vi "Y Scale Name Label Text Write.vi"(4 "error in (no error)":errorcluster, 5 "Value":string, 6 "Container State":T3, 7 "Display State In":T1) -> (0 "error out":errorcluster, 3 "Display State Out":T1)   [LabVIEW 2017, in "2D Feather.xctl"]
uses:
  <vilib>/Math Plots/2D Math Plots/2D Feather/2D Feather XCtrl/2D Feather.xctl
  <vilib>/_xctls/Container State.ctl
  <vilib>/Math Plots/2D Math Plots/2D Feather/2D Feather XCtrl/State.ctl
  <vilib>/Math Plots/2D Math Plots/2D Feather/2D Feather/2D Feather.lvclass
  e:/builds/penguin/labview/branches/2017/dev/dist/vi.lib/Math Plots/2D Math Plots/2D Plot/2D Plot/2D Plot.lvclass
  <vilib>/Math Plots/2D Math Plots/2D Plot/Action String/2DMathPlot Ctrl Act Queue.ctl
  <vilib>/Math Plots/2D Math Plots/2D Plot/Action String/2DMathPlot Ctrl Act Cluster.ctl
  <vilib>/Math Plots/2D Math Plots/2D Plot/Action String/2DMathPlot State Class.ctl
  <vilib>/Math Plots/2D Math Plots/2D Plot/2D Plot/2D Plot.lvclass
  <vilib>/_xctls/XControlSupport.lvlib
panel:
  # "Replace the Value Control below with a Control of desired type.\nDo not remove this Control or the others from the connector pane.\nDo not change the connector pane pattern.\nThe Value control should always be the third terminal from top on the input side in the connector pane."
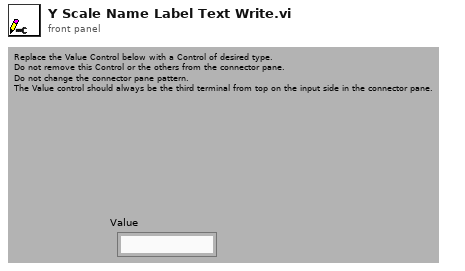
[diagram p1: front panel]
types:
  T1 = typedef "2D Feather.xctl/State.ctl" = cluster{"2D Feather.lvclass":refnum<class "2D Feather.lvclass">, "Control Ref Queue":T2, "Main Frame Color":u32, "Plot Legend Color":u32}
  T2 = typedef "2DMathPlot Ctrl Act Queue.ctl" = refnum<queue>
  T3 = typedef "XControlSupport.lvlib/Container State.ctl" = cluster{"Indicator?":bool, "Run Mode?":bool, " Refnum":refnum<vi>}
  T4 = typedef "2DMathPlot State Class.ctl" = enum16{"Update All (Undo)", "Update General", "Update Appearance", "Update Format", "Update Scale", "Update Marker", "Update Cursor", "None"}
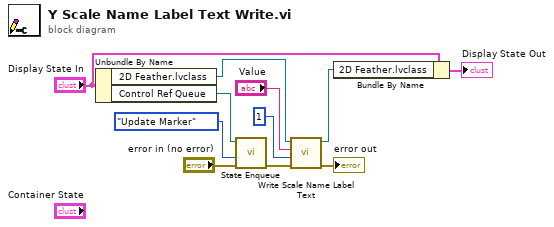
[diagram p0: block diagram]
diagram:
  n1 = Unbundle By Name("Display State In") -> ("2D Feather.lvclass"=w11:refnum<class "2D Feather.lvclass">, "Control Ref Queue"=w3:T2)
  n2 = call <vilib>:"State Enqueue.vi"("error in (no error)"="error in (no error)", "Display State Change Class"=2DMathPlot_State_Class."Update Marker", "Control Ref Queue"=w3) -> ("error out"=w1:errorcluster)  [unwired: 8 out]
  n3 = call <vilib>:"Write Scale Name Label Text.vi"("error in (no error)"=w1, "Index"=1, "Name Label Text"="Value", "2D Plot.lvclass in"=w11) -> ("error out"=→"error out":errorcluster, "2D Plot.lvclass out"=w10:refnum<class "2D Feather.lvclass">)  [unwired: 6 out]
  n4 = Bundle By Name(cluster="Display State In", "2D Feather.lvclass"=w10) -> (→"Display State Out":T1)
